vi "Set Visible Case.vi"(7 "Message Text":string, 8 "error in (no error)":errorcluster, 11 "CaseStructure in":refnum<vi>) -> (0 "error out":errorcluster)   [LabVIEW 2017, in "Open DQMH Request Message Diagram.lvlib"]
doc: "Changes the visible Case of the DQMH Module Main VI MHL."
uses:
  Open DQMH Request Message Diagram.lvlib
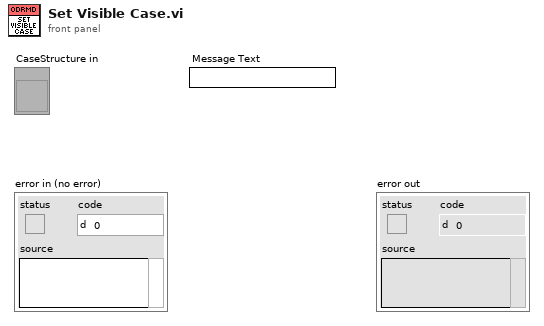
[diagram p1: front panel]
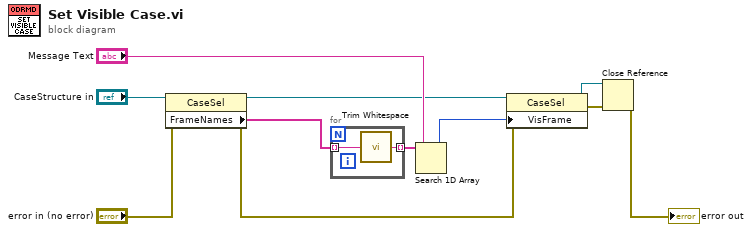
[diagram p0: block diagram]
diagram:
  n1 = property class="CaseSel"(reference="CaseStructure in", error in="error in (no error)") -> (reference out=w4:refnum<vi>, error out=w10:errorcluster, "FrameNames"=w5:string[])
  n2 = for {
    tunnel: [w13] -> w6 mode=indexing
    tunnel: w5 -> [w12] mode=indexing
    n3 = call <vilib>:"Trim Whitespace.vi"("string"=w12) -> ("trimmed string"=w13:string)  [unwired: 1 in]
  }
  n4 = Search 1D Array(1D array=w6, element="Message Text") -> (index of element=w9:i32)  [unwired: 1 in]
  n5 = property class="CaseSel"(reference=w4, error in=w10, "VisFrame"=w9) -> (reference out=w2:refnum<vi>, error out=w3:errorcluster)
  n6 = Close Reference(reference=w2, error in (no error)=w3) -> (error out=→"error out":errorcluster)
